vi "Get Type.vi"(8 "error in (no error)":errorcluster, 11 "SequenceFile in":refnum<class "SequenceFile.lvclass">) -> (0 "error out":errorcluster, 2 "Type":T1, 3 "SequenceFile out":refnum<class "SequenceFile.lvclass">)   [LabVIEW 2020, in "TSS.lvlib" / "SequenceFile.lvclass"]
uses:
  SequenceFile.lvclass
  Data Types/Sequence File Type.ctl
  SequenceFile.lvclass/SequenceFile.ctl
  TSS.lvlib
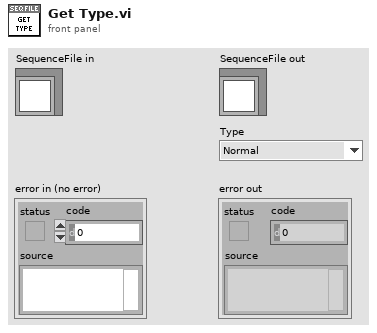
[diagram p1: front panel]
types:
  T1 = typedef "TSS.lvlib/Sequence File Type.ctl" = enum16{"Normal", "Model", "Front End Callbacks", "Station Callbacks", "Template"}
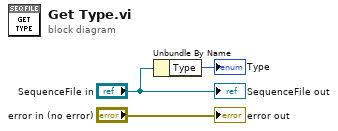
[diagram p0: block diagram]
diagram:
  n1 = Unbundle By Name("SequenceFile in") -> ("Type"=→"Type":T1)
  "error out" <- "error in (no error)"
  "SequenceFile out" <- "SequenceFile in"
